vi "KB-Laser move7-10.vi"(9 "Fitted Circle (Find Circular Edge 1)":T2 {"Average SNR (dB)" format="%.2f"; "Average Strength" format="%.2f"; "Roundness (Real-World)" format="%.2f"; "Radius (Real-World)" format="%.2f"; "Center (Real-World)"."Y" format="%.2f"; "Center (Real-World)"."X" format="%.2f"; "Radius (Pixels)" format="%.2f"; "Center (Pixels)"."Y" format="%.2f"; "Center (Pixels)"."X" format="%.2f"}, 10 "I roi":T1 {"Contours"."Type" items=["No Selection", "Point", "Line", "Rectangle", "Oval", "Polygon", "Freehand Region", "Annulus", "Unused2", "Unused3", "Broken Line", "Freehand Line", "Rotated Rectangle"]}, 11 "O roi":T1 {"Contours"."Type" items=["No Selection", "Point", "Line", "Rectangle", "Oval", "Polygon", "Freehand Region", "Annulus", "Unused2", "Unused3", "Broken Line", "Freehand Line", "Rotated Rectangle"]}) -> (2 "I roi Out":T1 {"Contours"."Type" items=["No Selection", "Point", "Line", "Rectangle", "Oval", "Polygon", "Freehand Region", "Annulus", "Unused2", "Unused3", "Broken Line", "Freehand Line", "Rotated Rectangle"]}, 3 "O roi Out":T1 {"Contours"."Type" items=["No Selection", "Point", "Line", "Rectangle", "Oval", "Polygon", "Freehand Region", "Annulus", "Unused2", "Unused3", "Broken Line", "Freehand Line", "Rotated Rectangle"]})   [LabVIEW 2015]
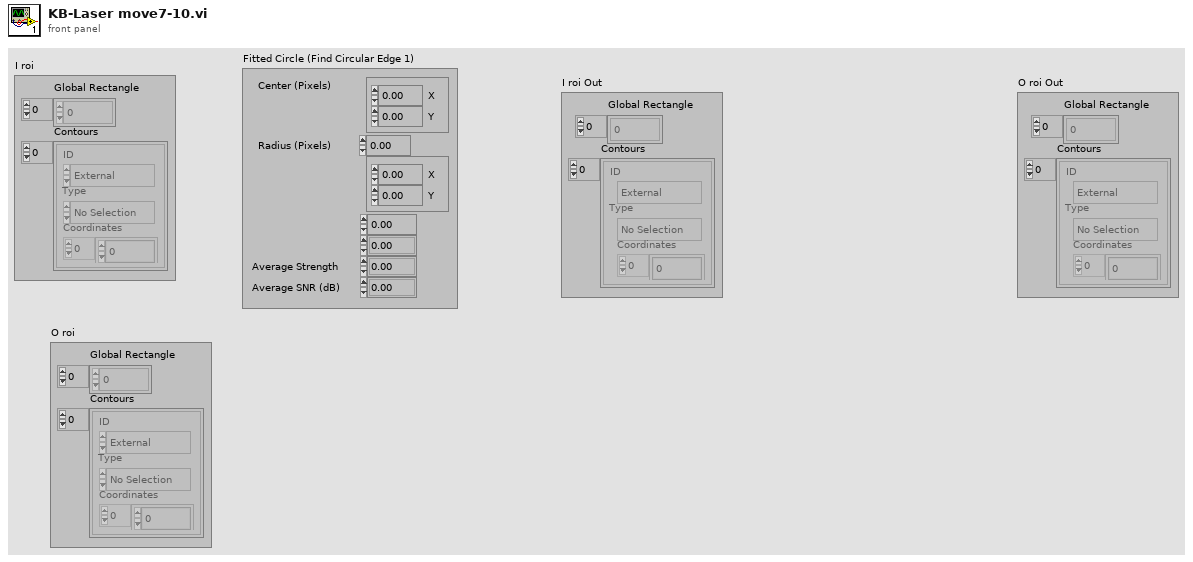
[diagram p1: front panel]
types:
  T1 = typedef "ROI Descriptor" = cluster{"Global Rectangle":i32[], "Contours":cluster{"ID":enum32{"External", "Internal"}, "Type":u32, "Coordinates":i32[]}[]}
  T2 = cluster{"Center (Pixels)":cluster{"X":sgl, "Y":sgl}, "Radius (Pixels)":dbl, "Center (Real-World)":cluster{"X":sgl, "Y":sgl}, "Radius (Real-World)":dbl, "Roundness (Real-World)":dbl, "Average Strength":dbl, "Average SNR (dB)":dbl}
  T3 = typedef "IMAQ Circle" = cluster{"Center X":i32, "Center Y":i32, "Inner Radius":i32, "Outer Radius":i32, "Start Angle":dbl, "End Angle":dbl}
  T4 = cluster{"ID":enum32{"External", "Internal"}, "Type":u32, "Coordinates":i32[]}[]
  T5 = cluster{"ID":enum32{"External", "Internal"}, "Type":u32, "Coordinates":i32[]}
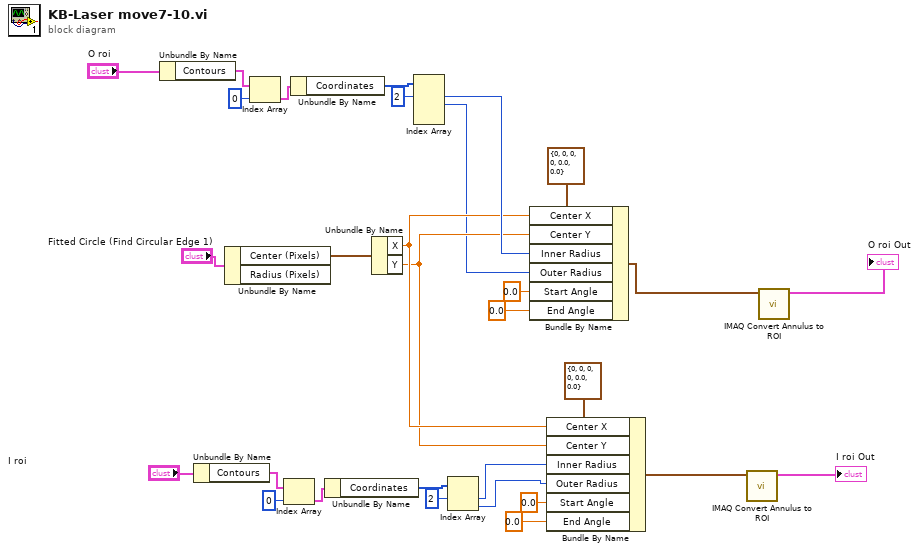
[diagram p0: block diagram]
diagram:
  n1 = Unbundle By Name("O roi") -> ("Contours"=w25:T4)
  n2 = Unbundle By Name("I roi") -> ("Contours"=w7:T4)
  n3 = Unbundle By Name("Fitted Circle (Find Circular Edge 1)") -> ("Center (Pixels)"=w29:cluster{"X":sgl, "Y":sgl})  [unwired: 1 out]
  n4 = Index Array(array=w25, index=0 ("索引")) -> (element=w23:T5)
  n5 = Index Array(array=w7, index=0 ("索引")) -> (element=w9:T5)
  n6 = Unbundle By Name(w23) -> ("Coordinates"=w22:i32[])
  n7 = Unbundle By Name(w9) -> ("Coordinates"=w10:i32[])
  n8 = Unbundle By Name(w29) -> ("X"=w13:sgl, "Y"=w12:sgl)
  n9 = Index Array(array=w22, index #1=2 ("索引")) -> (element #1=w20:i32, element #2=w1:i32)  [unwired: 3 in, 2 out]
  n10 = Index Array(array=w10, index #1=2 ("索引")) -> (element #1=w5:i32, element #2=w4:i32)  [unwired: 1 in]
  n11 = Bundle By Name(cluster=T3 {"Center X"=0, "Center Y"=0, "Inner Radius"=0, "Outer Radius"=0, "Start Angle"=0.0, "End Angle"=0.0} ("Annulus"), "Center X"=w13, "Center Y"=w12, "Inner Radius"=w20, "Outer Radius"=w1, "Start Angle"=0.0, "End Angle"=0.0) -> (w27:T3)
  n12 = Bundle By Name(cluster=T3 {"Center X"=0, "Center Y"=0, "Inner Radius"=0, "Outer Radius"=0, "Start Angle"=0.0, "End Angle"=0.0} ("Annulus"), "Center X"=w13, "Center Y"=w12, "Inner Radius"=w5, "Outer Radius"=w4, "Start Angle"=0.0, "End Angle"=0.0) -> (w3:T3)
  n13 = call "IMAQ Convert Annulus to ROI"("Annulus"=w3) -> ("ROI Descriptor"=→"I roi Out":T1)  [unwired: 8 in, 1 out]
  n14 = call "IMAQ Convert Annulus to ROI"("Annulus"=w27) -> ("ROI Descriptor"=→"O roi Out":T1)  [unwired: 8 in, 1 out]
